vi "RANGE Grab Bank Data.vi"(0 "DAQ Data In in":T4={"Meter 1"={"Meter Size"=0.0, "DAQ Output (Voltage)"=0.0, "Reference (Voltage)"=0.0, "Meter Present"=FALSE, "Meter Visa"="COM3", "Gas Type"="12", "SLPM Error @ Zero"=0.0, "Gas Mix Number"="", "Set STP Register"=FALSE, "Measurement Units"={"Software Rev"="", "Model Number"="", "Manufacturer Info"="", "Software Sub-Rev"="", "Board Rev"="", "Units of Measure Input"={"Abs. Pressure"="", "Gauge/Diff. Press."="", "Barometric Press."="", "Temperature"="", "Volume"="", "Mass"="", "Setpoint"="", "Valve Drive"="", "Totalizer"="", "Tot. Timer"="", "Tot. Avg. Flow"="", "Tot. Peak Flow"=""}}, "Data Frame Format"={"Absolute Pressure"=FALSE, "Gauge/Diff. Pressure"=FALSE, "Barometric Pressure"=FALSE, "Temperature"=FALSE, "Volumetric"=FALSE, "Mass"=FALSE, "Setpoint"=FALSE, "Valve Drive"=FALSE, "Totalizer"=FALSE, "Totalizer Timer"=FALSE, "Totalizer Average Flow"=FALSE, "Totalizer Peak Flow"=FALSE, "Gas Selected"=FALSE, "Tot. Timer Format"=0}}, "Meter 2"={"Meter Size"=0.0, "DAQ Output (Voltage)"=0.0, "Reference (Voltage)"=0.0, "Meter Present"=FALSE, "Meter Visa"="COM3", "Gas Type"="12", "SLPM Error @ Zero"=0.0, "Gas Mix Number"="", "Set STP Register"=FALSE, "Measurement Units"={"Software Rev"="", "Model Number"="", "Manufacturer Info"="", "Software Sub-Rev"="", "Board Rev"="", "Units of Measure Input"={"Abs. Pressure"="", "Gauge/Diff. Press."="", "Barometric Press."="", "Temperature"="", "Volume"="", "Mass"="", "Setpoint"="", "Valve Drive"="", "Totalizer"="", "Tot. Timer"="", "Tot. Avg. Flow"="", "Tot. Peak Flow"=""}}, "Data Frame Format"={"Absolute Pressure"=FALSE, "Gauge/Diff. Pressure"=FALSE, "Barometric Pressure"=FALSE, "Temperature"=FALSE, "Volumetric"=FALSE, "Mass"=FALSE, "Setpoint"=FALSE, "Valve Drive"=FALSE, "Totalizer"=FALSE, "Totalizer Timer"=FALSE, "Totalizer Average Flow"=FALSE, "Totalizer Peak Flow"=FALSE, "Gas Selected"=FALSE, "Tot. Timer Format"=0}}, "Meter 3"={"Meter Size"=0.0, "DAQ Output (Voltage)"=0.0, "Reference (Voltage)"=0.0, "Meter Present"=FALSE, "Meter Visa"="COM3", "Gas Type"="12", "SLPM Error @ Zero"=0.0, "Gas Mix Number"="", "Set STP Register"=FALSE, "Measurement Units"={"Software Rev"="", "Model Number"="", "Manufacturer Info"="", "Software Sub-Rev"="", "Board Rev"="", "Units of Measure Input"={"Abs. Pressure"="", "Gauge/Diff. Press."="", "Barometric Press."="", "Temperature"="", "Volume"="", "Mass"="", "Setpoint"="", "Valve Drive"="", "Totalizer"="", "Tot. Timer"="", "Tot. Avg. Flow"="", "Tot. Peak Flow"=""}}, "Data Frame Format"={"Absolute Pressure"=FALSE, "Gauge/Diff. Pressure"=FALSE, "Barometric Pressure"=FALSE, "Temperature"=FALSE, "Volumetric"=FALSE, "Mass"=FALSE, "Setpoint"=FALSE, "Valve Drive"=FALSE, "Totalizer"=FALSE, "Totalizer Timer"=FALSE, "Totalizer Average Flow"=FALSE, "Totalizer Peak Flow"=FALSE, "Gas Selected"=FALSE, "Tot. Timer Format"=0}}, "Meter 4"={"Meter Size"=0.0, "DAQ Output (Voltage)"=0.0, "Reference (Voltage)"=0.0, "Meter Present"=FALSE, "Meter Visa"="COM3", "Gas Type"="12", "SLPM Error @ Zero"=0.0, "Gas Mix Number"="", "Set STP Register"=FALSE, "Measurement Units"={"Software Rev"="", "Model Number"="", "Manufacturer Info"="", "Software Sub-Rev"="", "Board Rev"="", "Units of Measure Input"={"Abs. Pressure"="", "Gauge/Diff. Press."="", "Barometric Press."="", "Temperature"="", "Volume"="", "Mass"="", "Setpoint"="", "Valve Drive"="", "Totalizer"="", "Tot. Timer"="", "Tot. Avg. Flow"="", "Tot. Peak Flow"=""}}, "Data Frame Format"={"Absolute Pressure"=FALSE, "Gauge/Diff. Pressure"=FALSE, "Barometric Pressure"=FALSE, "Temperature"=FALSE, "Volumetric"=FALSE, "Mass"=FALSE, "Setpoint"=FALSE, "Valve Drive"=FALSE, "Totalizer"=FALSE, "Totalizer Timer"=FALSE, "Totalizer Average Flow"=FALSE, "Totalizer Peak Flow"=FALSE, "Gas Selected"=FALSE, "Tot. Timer Format"=0}}, "Meter 5"={"Meter Size"=0.0, "DAQ Output (Voltage)"=0.0, "Reference (Voltage)"=0.0, "Meter Present"=FALSE, "Meter Visa"="COM3", "Gas Type"="12", "SLPM Error @ Zero"=0.0, "Gas Mix Number"="", "Set STP Register"=FALSE, "Measurement Units"={"Software Rev"="", "Model Number"="", "Manufacturer Info"="", "Software Sub-Rev"="", "Board Rev"="", "Units of Measure Input"={"Abs. Pressure"="", "Gauge/Diff. Press."="", "Barometric Press."="", "Temperature"="", "Volume"="", "Mass"="", "Setpoint"="", "Valve Drive"="", "Totalizer"="", "Tot. Timer"="", "Tot. Avg. Flow"="", "Tot. Peak Flow"=""}}, "Data Frame Format"={"Absolute Pressure"=FALSE, "Gauge/Diff. Pressure"=FALSE, "Barometric Pressure"=FALSE, "Temperature"=FALSE, "Volumetric"=FALSE, "Mass"=FALSE, "Setpoint"=FALSE, "Valve Drive"=FALSE, "Totalizer"=FALSE, "Totalizer Timer"=FALSE, "Totalizer Average Flow"=FALSE, "Totalizer Peak Flow"=FALSE, "Gas Selected"=FALSE, "Tot. Timer Format"=0}}, "Meter 6"={"Meter Size"=0.0, "DAQ Output (Voltage)"=0.0, "Reference (Voltage)"=0.0, "Meter Present"=FALSE, "Meter Visa"="COM3", "Gas Type"="12", "SLPM Error @ Zero"=0.0, "Gas Mix Number"="", "Set STP Register"=FALSE, "Measurement Units"={"Software Rev"="", "Model Number"="", "Manufacturer Info"="", "Software Sub-Rev"="", "Board Rev"="", "Units of Measure Input"={"Abs. Pressure"="", "Gauge/Diff. Press."="", "Barometric Press."="", "Temperature"="", "Volume"="", "Mass"="", "Setpoint"="", "Valve Drive"="", "Totalizer"="", "Tot. Timer"="", "Tot. Avg. Flow"="", "Tot. Peak Flow"=""}}, "Data Frame Format"={"Absolute Pressure"=FALSE, "Gauge/Diff. Pressure"=FALSE, "Barometric Pressure"=FALSE, "Temperature"=FALSE, "Volumetric"=FALSE, "Mass"=FALSE, "Setpoint"=FALSE, "Valve Drive"=FALSE, "Totalizer"=FALSE, "Totalizer Timer"=FALSE, "Totalizer Average Flow"=FALSE, "Totalizer Peak Flow"=FALSE, "Gas Selected"=FALSE, "Tot. Timer Format"=0}}, "Meter Bank 1"={"Flow Rate (BTU/HR)"=0.0, "ANSI Average (BTU/HR)"=0.0, "Panel Data"={"Meter Type (Gas)"="", "Heating Value (BTU/ft³)"=0.0, "Ft³ / Hr (SCFH)"=0.0, "15 Second Average (BTU/HR)"=0.0, "30 Second Average (BTU/HR)"=0.0, "Mass Flow"=0.0, "Vol. Flow"=0.0, "Gas Temperature"=0.0, "Gas Pressure"=0.0, "Tot.Flow"=0.0}, "Meter ID"="", "ANSI Rate"={"Array 1"=[], "Array 3"=[], "Array 2"=[], "Start ANSI"=FALSE, "ANSI Start Time"=0.0, "Restart ANSI"=FALSE, "15 Min ANSI Avg (BTU/hr)"=0.0, "20 Min ANSI Avg (BTU/hr)"=0.0, "25 Min ANSI Avg (BTU/hr)"=0.0, "Absolute Pressure"=0.0, "Gas Temperature"=0.0, "Volumetric Flow Rate"=0.0, "Mass Flow Rate"=0.0, "Array 4"=[], "Array 5"=[], "Gas Rate"=0.0, "15 Min Pres Avg (PSIA)"=0.0, "20 Min Pres Avg (PSIA)"=0.0, "25 Min Pres Avg (PSIA)"=0.0, "15 Min Temp Avg (°F) "=0.0, "20 Min Temp Avg (°F)"=0.0, "25 Min Temp Avg (°F)"=0.0, "15 Min Uncorrected Avg (CFH)"=0.0, "20 Min Uncorrected Avg (CFH)"=0.0, "25 Min Uncorrected Avg (CFH)"=0.0, "15 Min Corrected Avg (SCFH)"=0.0, "20 Min Corrected Avg (SCFH)"=0.0, "25 Min Corrected Avg (SCFH)"=0.0, "15 Min Complete"=FALSE, "20 Min Complete"=FALSE, "25 Min Complete"=FALSE, "Heating Value (BTU/ft³)"=0.0, "CO CO2 15 Min"=[], "CO CO2 20 Min"=[], "CO CO2 25 Min"=[], "CO CO2 Real Time"=[]}}, "Meter Bank 2"={"Flow Rate (BTU/HR)"=0.0, "ANSI Average (BTU/HR)"=0.0, "Panel Data"={"Meter Type (Gas)"="", "Heating Value (BTU/ft³)"=0.0, "Ft³ / Hr (SCFH)"=0.0, "15 Second Average (BTU/HR)"=0.0, "30 Second Average (BTU/HR)"=0.0, "Mass Flow"=0.0, "Vol. Flow"=0.0, "Gas Temperature"=0.0, "Gas Pressure"=0.0, "Tot.Flow"=0.0}, "Meter ID"="", "ANSI Rate"={"Array 1"=[], "Array 3"=[], "Array 2"=[], "Start ANSI"=FALSE, "ANSI Start Time"=0.0, "Restart ANSI"=FALSE, "15 Min ANSI Avg (BTU/hr)"=0.0, "20 Min ANSI Avg (BTU/hr)"=0.0, "25 Min ANSI Avg (BTU/hr)"=0.0, "Absolute Pressure"=0.0, "Gas Temperature"=0.0, "Volumetric Flow Rate"=0.0, "Mass Flow Rate"=0.0, "Array 4"=[], "Array 5"=[], "Gas Rate"=0.0, "15 Min Pres Avg (PSIA)"=0.0, "20 Min Pres Avg (PSIA)"=0.0, "25 Min Pres Avg (PSIA)"=0.0, "15 Min Temp Avg (°F) "=0.0, "20 Min Temp Avg (°F)"=0.0, "25 Min Temp Avg (°F)"=0.0, "15 Min Uncorrected Avg (CFH)"=0.0, "20 Min Uncorrected Avg (CFH)"=0.0, "25 Min Uncorrected Avg (CFH)"=0.0, "15 Min Corrected Avg (SCFH)"=0.0, "20 Min Corrected Avg (SCFH)"=0.0, "25 Min Corrected Avg (SCFH)"=0.0, "15 Min Complete"=FALSE, "20 Min Complete"=FALSE, "25 Min Complete"=FALSE, "Heating Value (BTU/ft³)"=0.0, "CO CO2 15 Min"=[], "CO CO2 20 Min"=[], "CO CO2 25 Min"=[], "CO CO2 Real Time"=[]}}, "Meter Bank 3"={"Flow Rate (BTU/HR)"=0.0, "ANSI Average (BTU/HR)"=0.0, "Panel Data"={"Meter Type (Gas)"="", "Heating Value (BTU/ft³)"=0.0, "Ft³ / Hr (SCFH)"=0.0, "15 Second Average (BTU/HR)"=0.0, "30 Second Average (BTU/HR)"=0.0, "Mass Flow"=0.0, "Vol. Flow"=0.0, "Gas Temperature"=0.0, "Gas Pressure"=0.0, "Tot.Flow"=0.0}, "Meter ID"="", "ANSI Rate"={"Array 1"=[], "Array 3"=[], "Array 2"=[], "Start ANSI"=FALSE, "ANSI Start Time"=0.0, "Restart ANSI"=FALSE, "15 Min ANSI Avg (BTU/hr)"=0.0, "20 Min ANSI Avg (BTU/hr)"=0.0, "25 Min ANSI Avg (BTU/hr)"=0.0, "Absolute Pressure"=0.0, "Gas Temperature"=0.0, "Volumetric Flow Rate"=0.0, "Mass Flow Rate"=0.0, "Array 4"=[], "Array 5"=[], "Gas Rate"=0.0, "15 Min Pres Avg (PSIA)"=0.0, "20 Min Pres Avg (PSIA)"=0.0, "25 Min Pres Avg (PSIA)"=0.0, "15 Min Temp Avg (°F) "=0.0, "20 Min Temp Avg (°F)"=0.0, "25 Min Temp Avg (°F)"=0.0, "15 Min Uncorrected Avg (CFH)"=0.0, "20 Min Uncorrected Avg (CFH)"=0.0, "25 Min Uncorrected Avg (CFH)"=0.0, "15 Min Corrected Avg (SCFH)"=0.0, "20 Min Corrected Avg (SCFH)"=0.0, "25 Min Corrected Avg (SCFH)"=0.0, "15 Min Complete"=FALSE, "20 Min Complete"=FALSE, "25 Min Complete"=FALSE, "Heating Value (BTU/ft³)"=0.0, "CO CO2 15 Min"=[], "CO CO2 20 Min"=[], "CO CO2 25 Min"=[], "CO CO2 Real Time"=[]}}, "Threshold Voltage (NI DAQ)"=0.0, "Use RS232 Data Collection"=FALSE, "Use Auto Switching"=FALSE}, 1 "Meter Number":T13, 2 "Tot.Flow (Liters) Bank 2":dbl, 3 "Use Mass Flow Unit Converter?":bool, 5 "Meter Select":T3, 7 "Tot.Flow (Liters) Bank 1":dbl, 9 "Meter Select 2":T1, 11 "error in (no error)":errorcluster, 12 "Meter Select 3":T2, 13 "Tot.Flow (Liters) Bank 3":dbl) -> (4 "DAQ Data In out":T4={"Meter 1"={"Meter Size"=0.0, "DAQ Output (Voltage)"=0.0, "Reference (Voltage)"=0.0, "Meter Present"=FALSE, "Meter Visa"="COM3", "Gas Type"="12", "SLPM Error @ Zero"=0.0, "Gas Mix Number"="", "Set STP Register"=FALSE, "Measurement Units"={"Software Rev"="", "Model Number"="", "Manufacturer Info"="", "Software Sub-Rev"="", "Board Rev"="", "Units of Measure Input"={"Abs. Pressure"="", "Gauge/Diff. Press."="", "Barometric Press."="", "Temperature"="", "Volume"="", "Mass"="", "Setpoint"="", "Valve Drive"="", "Totalizer"="", "Tot. Timer"="", "Tot. Avg. Flow"="", "Tot. Peak Flow"=""}}, "Data Frame Format"={"Absolute Pressure"=FALSE, "Gauge/Diff. Pressure"=FALSE, "Barometric Pressure"=FALSE, "Temperature"=FALSE, "Volumetric"=FALSE, "Mass"=FALSE, "Setpoint"=FALSE, "Valve Drive"=FALSE, "Totalizer"=FALSE, "Totalizer Timer"=FALSE, "Totalizer Average Flow"=FALSE, "Totalizer Peak Flow"=FALSE, "Gas Selected"=FALSE, "Tot. Timer Format"=0}}, "Meter 2"={"Meter Size"=0.0, "DAQ Output (Voltage)"=0.0, "Reference (Voltage)"=0.0, "Meter Present"=FALSE, "Meter Visa"="COM3", "Gas Type"="12", "SLPM Error @ Zero"=0.0, "Gas Mix Number"="", "Set STP Register"=FALSE, "Measurement Units"={"Software Rev"="", "Model Number"="", "Manufacturer Info"="", "Software Sub-Rev"="", "Board Rev"="", "Units of Measure Input"={"Abs. Pressure"="", "Gauge/Diff. Press."="", "Barometric Press."="", "Temperature"="", "Volume"="", "Mass"="", "Setpoint"="", "Valve Drive"="", "Totalizer"="", "Tot. Timer"="", "Tot. Avg. Flow"="", "Tot. Peak Flow"=""}}, "Data Frame Format"={"Absolute Pressure"=FALSE, "Gauge/Diff. Pressure"=FALSE, "Barometric Pressure"=FALSE, "Temperature"=FALSE, "Volumetric"=FALSE, "Mass"=FALSE, "Setpoint"=FALSE, "Valve Drive"=FALSE, "Totalizer"=FALSE, "Totalizer Timer"=FALSE, "Totalizer Average Flow"=FALSE, "Totalizer Peak Flow"=FALSE, "Gas Selected"=FALSE, "Tot. Timer Format"=0}}, "Meter 3"={"Meter Size"=0.0, "DAQ Output (Voltage)"=0.0, "Reference (Voltage)"=0.0, "Meter Present"=FALSE, "Meter Visa"="COM3", "Gas Type"="12", "SLPM Error @ Zero"=0.0, "Gas Mix Number"="", "Set STP Register"=FALSE, "Measurement Units"={"Software Rev"="", "Model Number"="", "Manufacturer Info"="", "Software Sub-Rev"="", "Board Rev"="", "Units of Measure Input"={"Abs. Pressure"="", "Gauge/Diff. Press."="", "Barometric Press."="", "Temperature"="", "Volume"="", "Mass"="", "Setpoint"="", "Valve Drive"="", "Totalizer"="", "Tot. Timer"="", "Tot. Avg. Flow"="", "Tot. Peak Flow"=""}}, "Data Frame Format"={"Absolute Pressure"=FALSE, "Gauge/Diff. Pressure"=FALSE, "Barometric Pressure"=FALSE, "Temperature"=FALSE, "Volumetric"=FALSE, "Mass"=FALSE, "Setpoint"=FALSE, "Valve Drive"=FALSE, "Totalizer"=FALSE, "Totalizer Timer"=FALSE, "Totalizer Average Flow"=FALSE, "Totalizer Peak Flow"=FALSE, "Gas Selected"=FALSE, "Tot. Timer Format"=0}}, "Meter 4"={"Meter Size"=0.0, "DAQ Output (Voltage)"=0.0, "Reference (Voltage)"=0.0, "Meter Present"=FALSE, "Meter Visa"="COM3", "Gas Type"="12", "SLPM Error @ Zero"=0.0, "Gas Mix Number"="", "Set STP Register"=FALSE, "Measurement Units"={"Software Rev"="", "Model Number"="", "Manufacturer Info"="", "Software Sub-Rev"="", "Board Rev"="", "Units of Measure Input"={"Abs. Pressure"="", "Gauge/Diff. Press."="", "Barometric Press."="", "Temperature"="", "Volume"="", "Mass"="", "Setpoint"="", "Valve Drive"="", "Totalizer"="", "Tot. Timer"="", "Tot. Avg. Flow"="", "Tot. Peak Flow"=""}}, "Data Frame Format"={"Absolute Pressure"=FALSE, "Gauge/Diff. Pressure"=FALSE, "Barometric Pressure"=FALSE, "Temperature"=FALSE, "Volumetric"=FALSE, "Mass"=FALSE, "Setpoint"=FALSE, "Valve Drive"=FALSE, "Totalizer"=FALSE, "Totalizer Timer"=FALSE, "Totalizer Average Flow"=FALSE, "Totalizer Peak Flow"=FALSE, "Gas Selected"=FALSE, "Tot. Timer Format"=0}}, "Meter 5"={"Meter Size"=0.0, "DAQ Output (Voltage)"=0.0, "Reference (Voltage)"=0.0, "Meter Present"=FALSE, "Meter Visa"="COM3", "Gas Type"="12", "SLPM Error @ Zero"=0.0, "Gas Mix Number"="", "Set STP Register"=FALSE, "Measurement Units"={"Software Rev"="", "Model Number"="", "Manufacturer Info"="", "Software Sub-Rev"="", "Board Rev"="", "Units of Measure Input"={"Abs. Pressure"="", "Gauge/Diff. Press."="", "Barometric Press."="", "Temperature"="", "Volume"="", "Mass"="", "Setpoint"="", "Valve Drive"="", "Totalizer"="", "Tot. Timer"="", "Tot. Avg. Flow"="", "Tot. Peak Flow"=""}}, "Data Frame Format"={"Absolute Pressure"=FALSE, "Gauge/Diff. Pressure"=FALSE, "Barometric Pressure"=FALSE, "Temperature"=FALSE, "Volumetric"=FALSE, "Mass"=FALSE, "Setpoint"=FALSE, "Valve Drive"=FALSE, "Totalizer"=FALSE, "Totalizer Timer"=FALSE, "Totalizer Average Flow"=FALSE, "Totalizer Peak Flow"=FALSE, "Gas Selected"=FALSE, "Tot. Timer Format"=0}}, "Meter 6"={"Meter Size"=0.0, "DAQ Output (Voltage)"=0.0, "Reference (Voltage)"=0.0, "Meter Present"=FALSE, "Meter Visa"="COM3", "Gas Type"="12", "SLPM Error @ Zero"=0.0, "Gas Mix Number"="", "Set STP Register"=FALSE, "Measurement Units"={"Software Rev"="", "Model Number"="", "Manufacturer Info"="", "Software Sub-Rev"="", "Board Rev"="", "Units of Measure Input"={"Abs. Pressure"="", "Gauge/Diff. Press."="", "Barometric Press."="", "Temperature"="", "Volume"="", "Mass"="", "Setpoint"="", "Valve Drive"="", "Totalizer"="", "Tot. Timer"="", "Tot. Avg. Flow"="", "Tot. Peak Flow"=""}}, "Data Frame Format"={"Absolute Pressure"=FALSE, "Gauge/Diff. Pressure"=FALSE, "Barometric Pressure"=FALSE, "Temperature"=FALSE, "Volumetric"=FALSE, "Mass"=FALSE, "Setpoint"=FALSE, "Valve Drive"=FALSE, "Totalizer"=FALSE, "Totalizer Timer"=FALSE, "Totalizer Average Flow"=FALSE, "Totalizer Peak Flow"=FALSE, "Gas Selected"=FALSE, "Tot. Timer Format"=0}}, "Meter Bank 1"={"Flow Rate (BTU/HR)"=0.0, "ANSI Average (BTU/HR)"=0.0, "Panel Data"={"Meter Type (Gas)"="", "Heating Value (BTU/ft³)"=0.0, "Ft³ / Hr (SCFH)"=0.0, "15 Second Average (BTU/HR)"=0.0, "30 Second Average (BTU/HR)"=0.0, "Mass Flow"=0.0, "Vol. Flow"=0.0, "Gas Temperature"=0.0, "Gas Pressure"=0.0, "Tot.Flow"=0.0}, "Meter ID"="", "ANSI Rate"={"Array 1"=[], "Array 3"=[], "Array 2"=[], "Start ANSI"=FALSE, "ANSI Start Time"=0.0, "Restart ANSI"=FALSE, "15 Min ANSI Avg (BTU/hr)"=0.0, "20 Min ANSI Avg (BTU/hr)"=0.0, "25 Min ANSI Avg (BTU/hr)"=0.0, "Absolute Pressure"=0.0, "Gas Temperature"=0.0, "Volumetric Flow Rate"=0.0, "Mass Flow Rate"=0.0, "Array 4"=[], "Array 5"=[], "Gas Rate"=0.0, "15 Min Pres Avg (PSIA)"=0.0, "20 Min Pres Avg (PSIA)"=0.0, "25 Min Pres Avg (PSIA)"=0.0, "15 Min Temp Avg (°F) "=0.0, "20 Min Temp Avg (°F)"=0.0, "25 Min Temp Avg (°F)"=0.0, "15 Min Uncorrected Avg (CFH)"=0.0, "20 Min Uncorrected Avg (CFH)"=0.0, "25 Min Uncorrected Avg (CFH)"=0.0, "15 Min Corrected Avg (SCFH)"=0.0, "20 Min Corrected Avg (SCFH)"=0.0, "25 Min Corrected Avg (SCFH)"=0.0, "15 Min Complete"=FALSE, "20 Min Complete"=FALSE, "25 Min Complete"=FALSE, "Heating Value (BTU/ft³)"=0.0, "CO CO2 15 Min"=[], "CO CO2 20 Min"=[], "CO CO2 25 Min"=[], "CO CO2 Real Time"=[]}}, "Meter Bank 2"={"Flow Rate (BTU/HR)"=0.0, "ANSI Average (BTU/HR)"=0.0, "Panel Data"={"Meter Type (Gas)"="", "Heating Value (BTU/ft³)"=0.0, "Ft³ / Hr (SCFH)"=0.0, "15 Second Average (BTU/HR)"=0.0, "30 Second Average (BTU/HR)"=0.0, "Mass Flow"=0.0, "Vol. Flow"=0.0, "Gas Temperature"=0.0, "Gas Pressure"=0.0, "Tot.Flow"=0.0}, "Meter ID"="", "ANSI Rate"={"Array 1"=[], "Array 3"=[], "Array 2"=[], "Start ANSI"=FALSE, "ANSI Start Time"=0.0, "Restart ANSI"=FALSE, "15 Min ANSI Avg (BTU/hr)"=0.0, "20 Min ANSI Avg (BTU/hr)"=0.0, "25 Min ANSI Avg (BTU/hr)"=0.0, "Absolute Pressure"=0.0, "Gas Temperature"=0.0, "Volumetric Flow Rate"=0.0, "Mass Flow Rate"=0.0, "Array 4"=[], "Array 5"=[], "Gas Rate"=0.0, "15 Min Pres Avg (PSIA)"=0.0, "20 Min Pres Avg (PSIA)"=0.0, "25 Min Pres Avg (PSIA)"=0.0, "15 Min Temp Avg (°F) "=0.0, "20 Min Temp Avg (°F)"=0.0, "25 Min Temp Avg (°F)"=0.0, "15 Min Uncorrected Avg (CFH)"=0.0, "20 Min Uncorrected Avg (CFH)"=0.0, "25 Min Uncorrected Avg (CFH)"=0.0, "15 Min Corrected Avg (SCFH)"=0.0, "20 Min Corrected Avg (SCFH)"=0.0, "25 Min Corrected Avg (SCFH)"=0.0, "15 Min Complete"=FALSE, "20 Min Complete"=FALSE, "25 Min Complete"=FALSE, "Heating Value (BTU/ft³)"=0.0, "CO CO2 15 Min"=[], "CO CO2 20 Min"=[], "CO CO2 25 Min"=[], "CO CO2 Real Time"=[]}}, "Meter Bank 3"={"Flow Rate (BTU/HR)"=0.0, "ANSI Average (BTU/HR)"=0.0, "Panel Data"={"Meter Type (Gas)"="", "Heating Value (BTU/ft³)"=0.0, "Ft³ / Hr (SCFH)"=0.0, "15 Second Average (BTU/HR)"=0.0, "30 Second Average (BTU/HR)"=0.0, "Mass Flow"=0.0, "Vol. Flow"=0.0, "Gas Temperature"=0.0, "Gas Pressure"=0.0, "Tot.Flow"=0.0}, "Meter ID"="", "ANSI Rate"={"Array 1"=[], "Array 3"=[], "Array 2"=[], "Start ANSI"=FALSE, "ANSI Start Time"=0.0, "Restart ANSI"=FALSE, "15 Min ANSI Avg (BTU/hr)"=0.0, "20 Min ANSI Avg (BTU/hr)"=0.0, "25 Min ANSI Avg (BTU/hr)"=0.0, "Absolute Pressure"=0.0, "Gas Temperature"=0.0, "Volumetric Flow Rate"=0.0, "Mass Flow Rate"=0.0, "Array 4"=[], "Array 5"=[], "Gas Rate"=0.0, "15 Min Pres Avg (PSIA)"=0.0, "20 Min Pres Avg (PSIA)"=0.0, "25 Min Pres Avg (PSIA)"=0.0, "15 Min Temp Avg (°F) "=0.0, "20 Min Temp Avg (°F)"=0.0, "25 Min Temp Avg (°F)"=0.0, "15 Min Uncorrected Avg (CFH)"=0.0, "20 Min Uncorrected Avg (CFH)"=0.0, "25 Min Uncorrected Avg (CFH)"=0.0, "15 Min Corrected Avg (SCFH)"=0.0, "20 Min Corrected Avg (SCFH)"=0.0, "25 Min Corrected Avg (SCFH)"=0.0, "15 Min Complete"=FALSE, "20 Min Complete"=FALSE, "25 Min Complete"=FALSE, "Heating Value (BTU/ft³)"=0.0, "CO CO2 15 Min"=[], "CO CO2 20 Min"=[], "CO CO2 25 Min"=[], "CO CO2 Real Time"=[]}}, "Threshold Voltage (NI DAQ)"=0.0, "Use RS232 Data Collection"=FALSE, "Use Auto Switching"=FALSE}, 15 "error out":errorcluster)   [LabVIEW 2023]
uses:
  Type Definitions/RANGE DAQ Data Four Meters.ctl
  Type Definitions/RANGE DAQ Data.ctl
  Drivers/Omega FMA-1600A Series Gas Flow Meter/Type Definitions/FMA1600A Gas Type.ctl
  Drivers/Omega FMA-1600A Series Gas Flow Meter/Type Definitions/FMA1600A Units String.ctl
  Drivers/Alicat Gas Meter Driver/Sub-VIs/Units of Measure.ctl
  Drivers/Alicat Gas Meter Driver/Sub-VIs/Data Frame.ctl
  Type Definitions/RANGE GAS Data.ctl
  Type Definitions/RANGE Panel Data.ctl
  Type Definitions/RANGE ANSI Rate.ctl
  Type Definitions/Range Meter Bank.ctl
  Type Definitions/RANGE Meter Selector 1-2.ctl
  Type Definitions/RANGE Meter Selector 5-6.ctl
  Type Definitions/RANGE Meter Selector 3-4.ctl
panel:
  out "x-y 2":dbl
  out "x-y":dbl
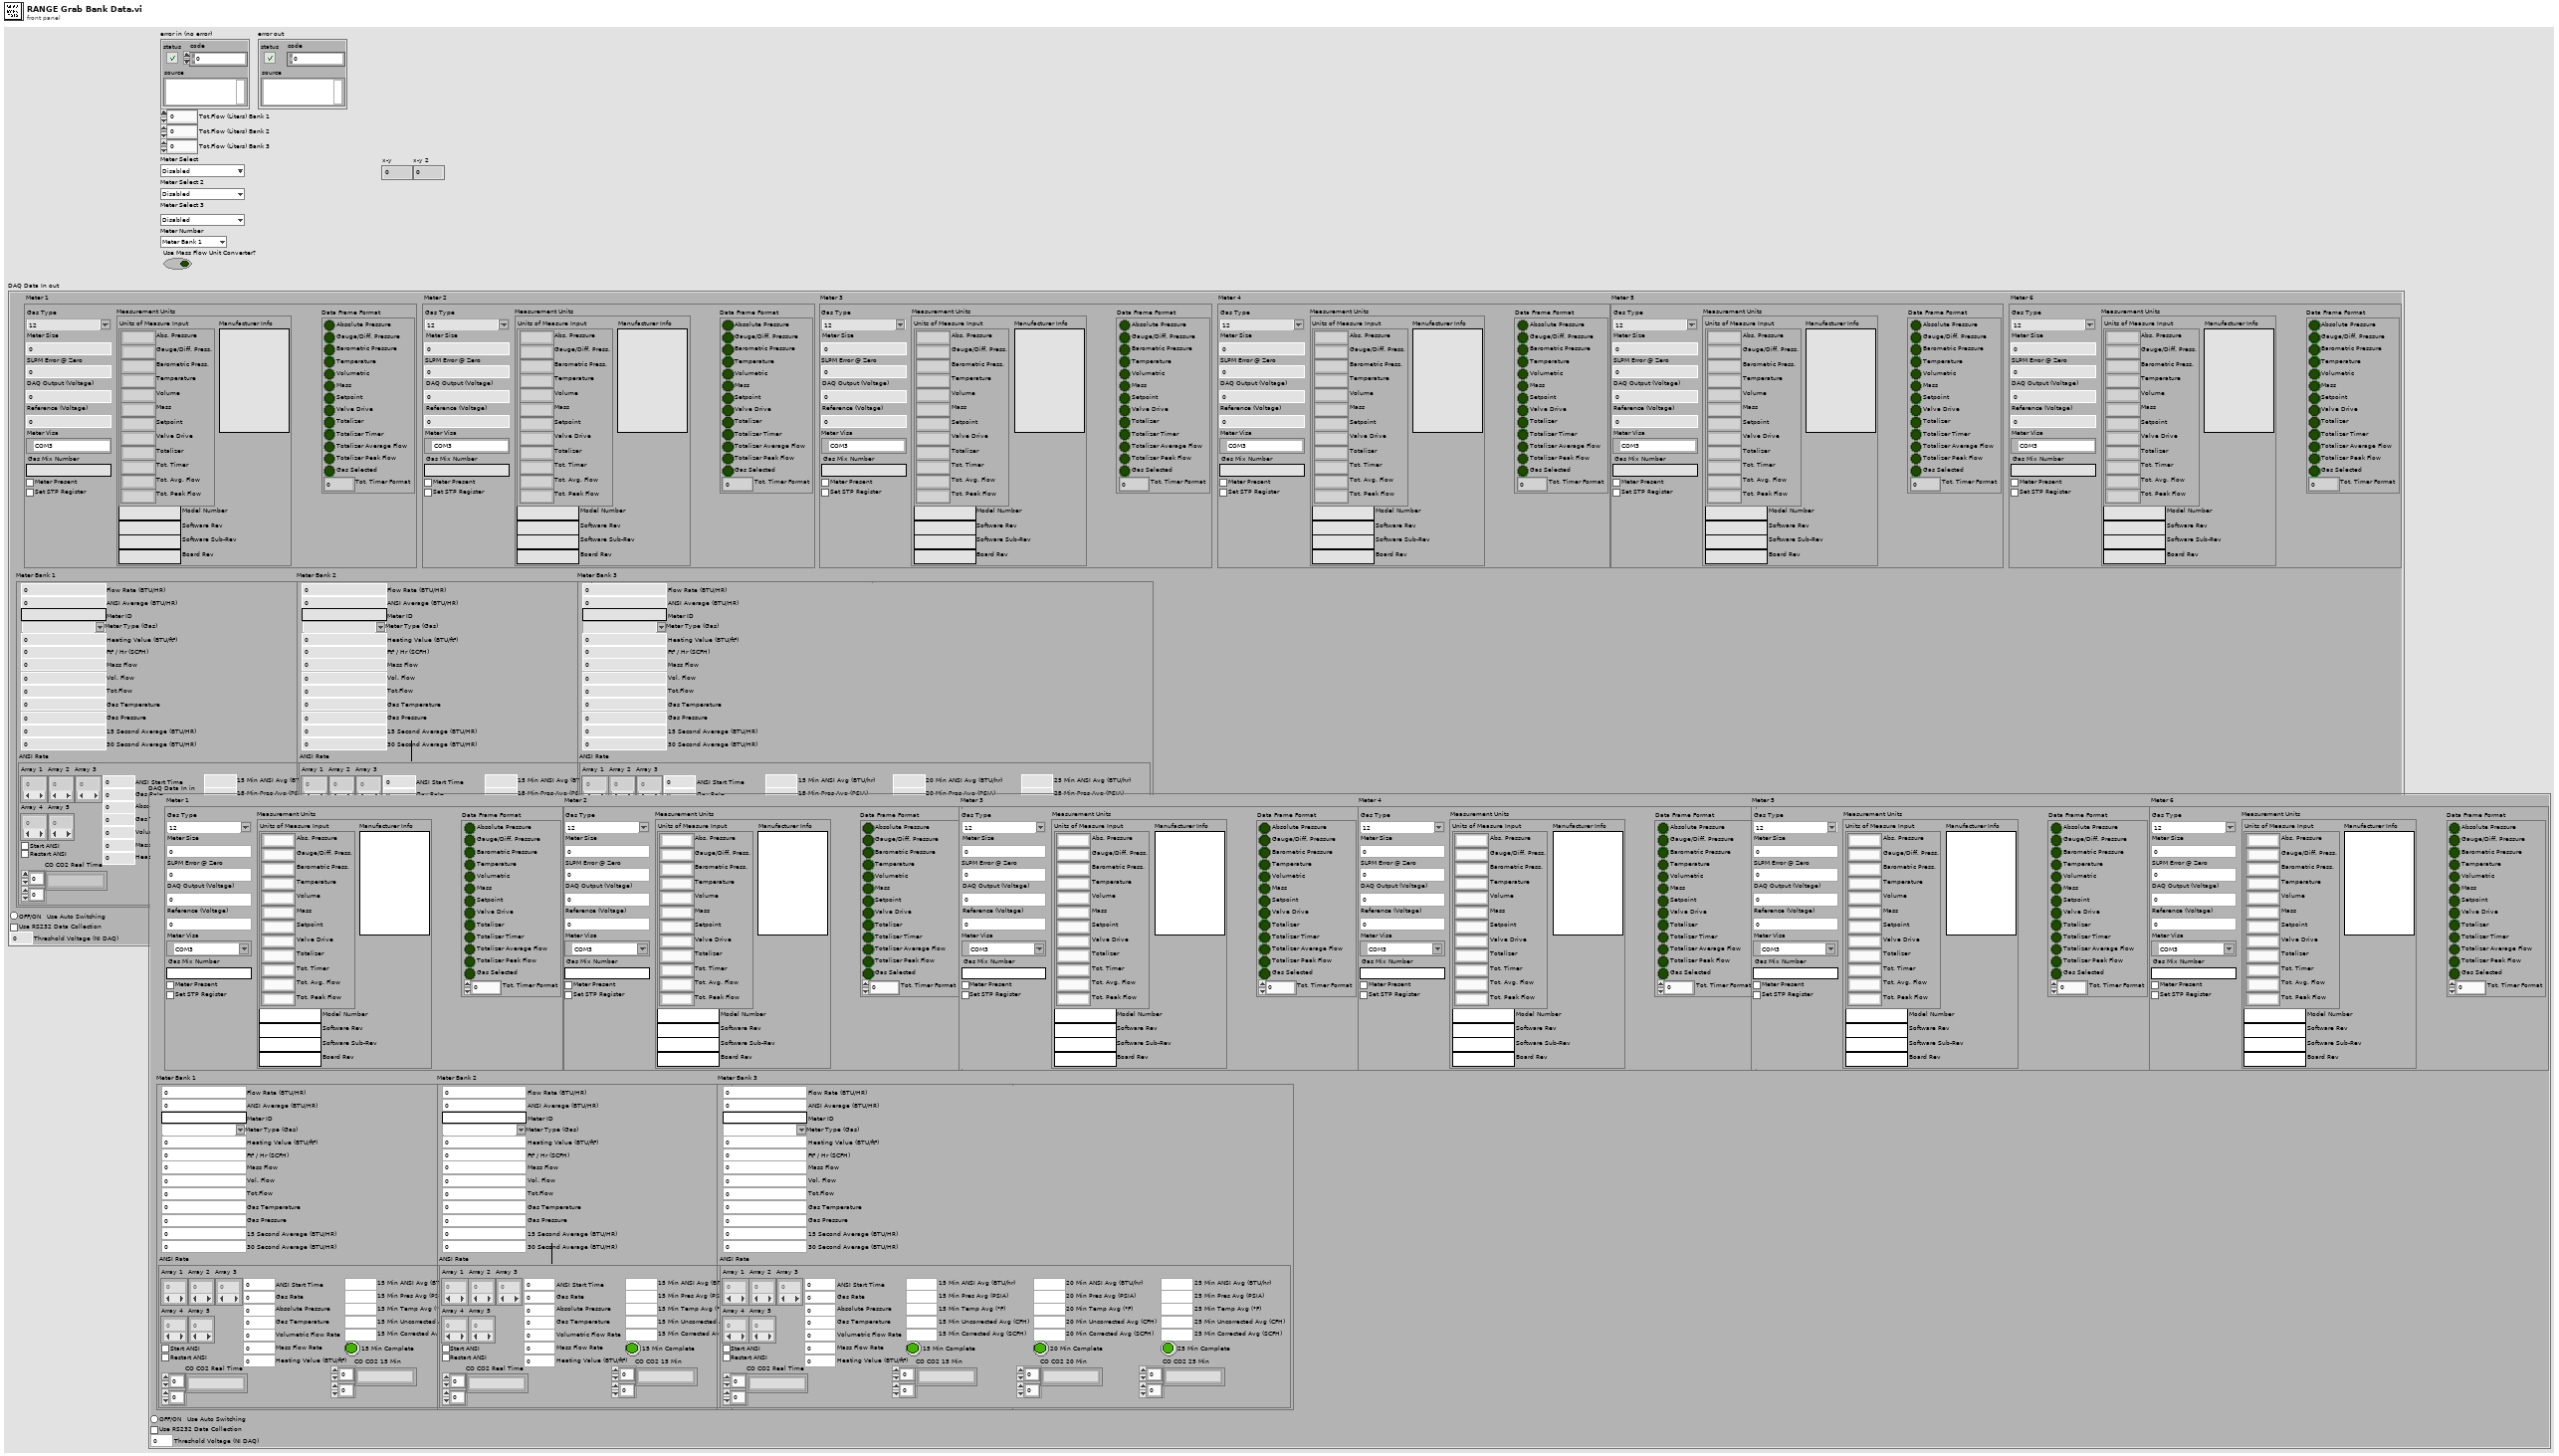
[diagram p1: front panel]
types:
  T1 = typedef "RANGE Meter Selector 3-4.ctl" = enum16{"Disabled", "Meter 3", "Meter 4", "Auto"}
  T2 = typedef "RANGE Meter Selector 5-6.ctl" = enum16{"Disabled", "Meter 5", "Meter 6", "Auto"}
  T3 = typedef "RANGE Meter Selector 1-2.ctl" = enum16{"Disabled", "Meter 1", "Meter 2", "Auto"}
  T4 = typedef "RANGE DAQ Data Four Meters.ctl" = cluster{"Meter 1":T5, "Meter 2":T5, "Meter 3":T5, "Meter 4":T5, "Meter 5":T5, "Meter 6":T5, "Meter Bank 1":T10, "Meter Bank 2":T10, "Meter Bank 3":T10, "Threshold Voltage (NI DAQ)":dbl, "Use RS232 Data Collection":bool, "Use Auto Switching":bool}
  T5 = typedef "RANGE DAQ Data.ctl" = cluster{"Meter Size":dbl, "DAQ Output (Voltage)":dbl, "Reference (Voltage)":dbl, "Meter Present":bool, "Meter Visa":refnum<visa-resource-name>, "Gas Type":T6, "SLPM Error @ Zero":dbl, "Gas Mix Number":string, "Set STP Register":bool, "Measurement Units":T7, "Data Frame Format":T9}
  T6 = typedef "FMA1600A Gas Type.ctl" = string
  T7 = typedef "FMA1600A Units String.ctl" = cluster{"Software Rev":string, "Model Number":string, "Manufacturer Info":string, "Software Sub-Rev":string, "Board Rev":string, "Units of Measure Input":T8}
  T8 = typedef "Units of Measure.ctl" = cluster{"Abs. Pressure":string, "Gauge/Diff. Press.":string, "Barometric Press.":string, "Temperature":string, "Volume":string, "Mass":string, "Setpoint":string, "Valve Drive":string, "Totalizer":string, "Tot. Timer":string, "Tot. Avg. Flow":string, "Tot. Peak Flow":string}
  T9 = typedef "Data Frame.ctl" = cluster{"Absolute Pressure":bool, "Gauge/Diff. Pressure":bool, "Barometric Pressure":bool, "Temperature":bool, "Volumetric":bool, "Mass":bool, "Setpoint":bool, "Valve Drive":bool, "Totalizer":bool, "Totalizer Timer":bool, "Totalizer Average Flow":bool, "Totalizer Peak Flow":bool, "Gas Selected":bool, "Tot. Timer Format":u16}
  T10 = typedef "RANGE GAS Data.ctl" = cluster{"Flow Rate (BTU/HR)":dbl, "ANSI Average (BTU/HR)":dbl, "Panel Data":T11, "Meter ID":string, "ANSI Rate":T12}
  T11 = typedef "RANGE Panel Data.ctl" = cluster{"Meter Type (Gas)":T6, "Heating Value (BTU/ft³)":dbl, "Ft³ / Hr (SCFH)":dbl, "15 Second Average (BTU/HR)":dbl, "30 Second Average (BTU/HR)":dbl, "Mass Flow":dbl, "Vol. Flow":dbl, "Gas Temperature":dbl, "Gas Pressure":dbl, "Tot.Flow":dbl}
  T12 = typedef "RANGE ANSI Rate.ctl" = cluster{"Array 1":dbl[], "Array 3":dbl[], "Array 2":dbl[], "Start ANSI":bool, "ANSI Start Time":dbl, "Restart ANSI":bool, "15 Min ANSI Avg (BTU/hr)":dbl, "20 Min ANSI Avg (BTU/hr)":dbl, "25 Min ANSI Avg (BTU/hr)":dbl, "Absolute Pressure":dbl, "Gas Temperature":dbl, "Volumetric Flow Rate":dbl, "Mass Flow Rate":dbl, "Array 4":dbl[], "Array 5":dbl[], "Gas Rate":dbl, "15 Min Pres Avg (PSIA)":dbl, "20 Min Pres Avg (PSIA)":dbl, "25 Min Pres Avg (PSIA)":dbl, "15 Min Temp Avg (°F) ":dbl, "20 Min Temp Avg (°F)":dbl, "25 Min Temp Avg (°F)":dbl, "15 Min Uncorrected Avg (CFH)":dbl, "20 Min Uncorrected Avg (CFH)":dbl, "25 Min Uncorrected Avg (CFH)":dbl, "15 Min Corrected Avg (SCFH)":dbl, "20 Min Corrected Avg (SCFH)":dbl, "25 Min Corrected Avg (SCFH)":dbl, "15 Min Complete":bool, "20 Min Complete":bool, "25 Min Complete":bool, "Heating Value (BTU/ft³)":dbl, "CO CO2 15 Min":string[][], "CO CO2 20 Min":string[][], "CO CO2 25 Min":string[][], "CO CO2 Real Time":string[][]}
  T13 = typedef "Range Meter Bank.ctl" = enum16{"Meter Bank 1", "Meter Bank 2", "Meter Bank 3"}
  T14 = typedef "Data Cluster.ctl" = cluster{"Absolute Pressure":dbl, "Gauge/Diff. Pressure":dbl, "Barometric Pressure":dbl, "Temperature":dbl, "Volumetric Flow":dbl, "Mass Flow":dbl, "Setpoint":dbl, "Valve Drive":dbl, "Totalizer":dbl, "[hr]":dbl, "[min]":dbl, "[sec]":dbl, "Totalizer Average Flow":dbl, "Totalizer Peak Flow":dbl, "Gas selected":string}
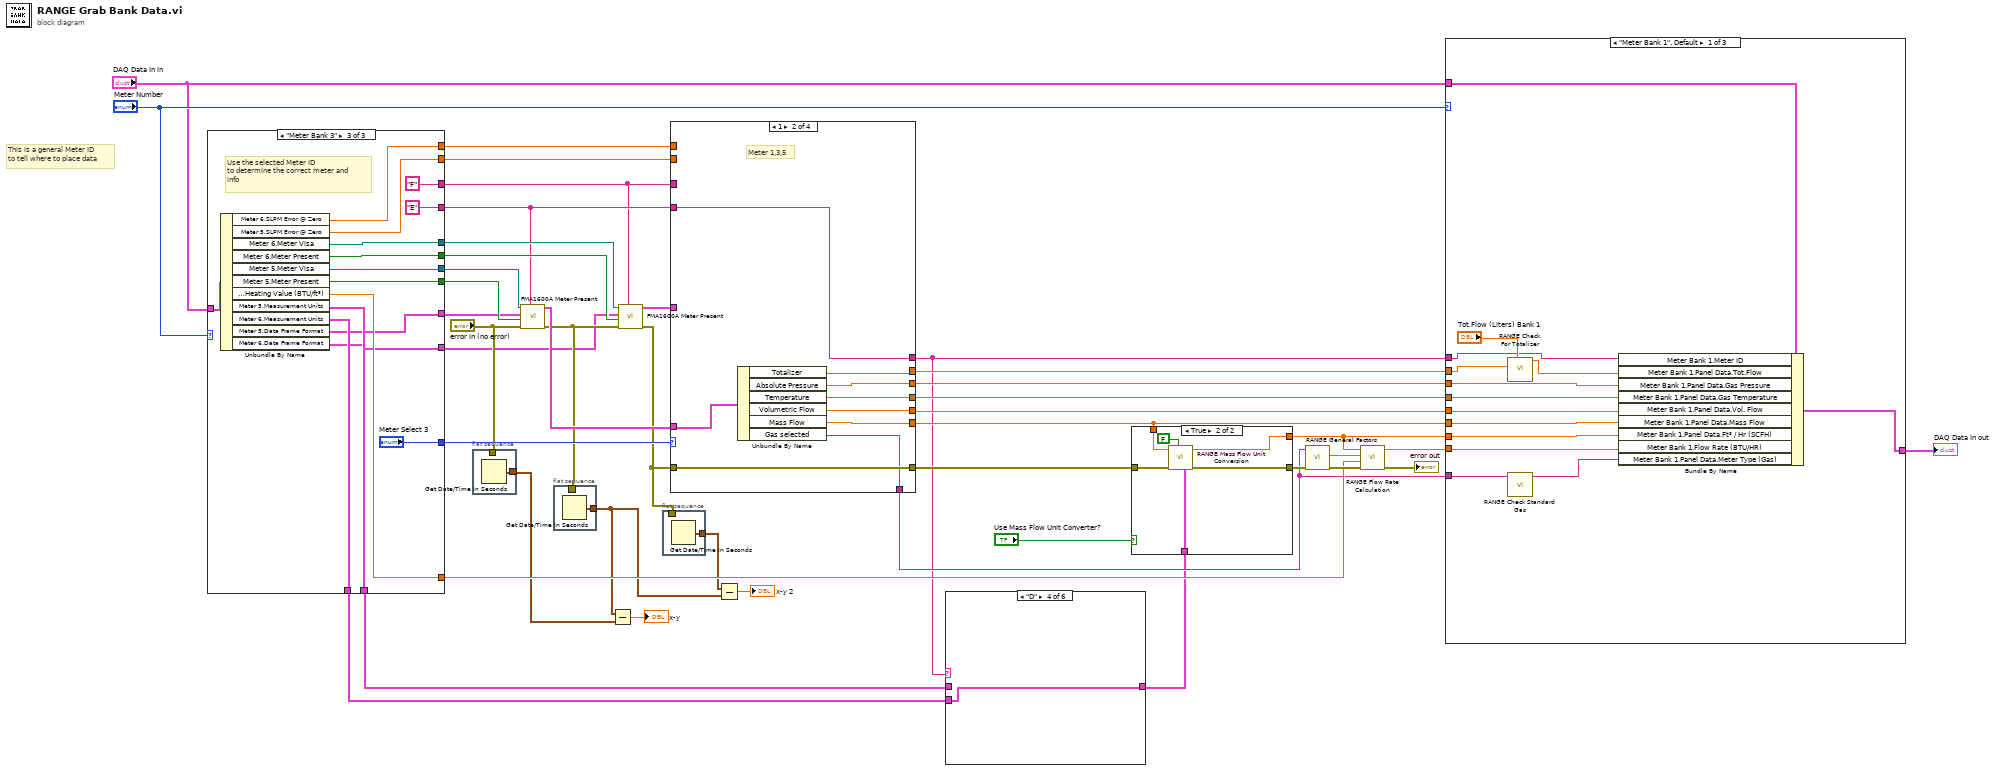
[diagram p0: block diagram]
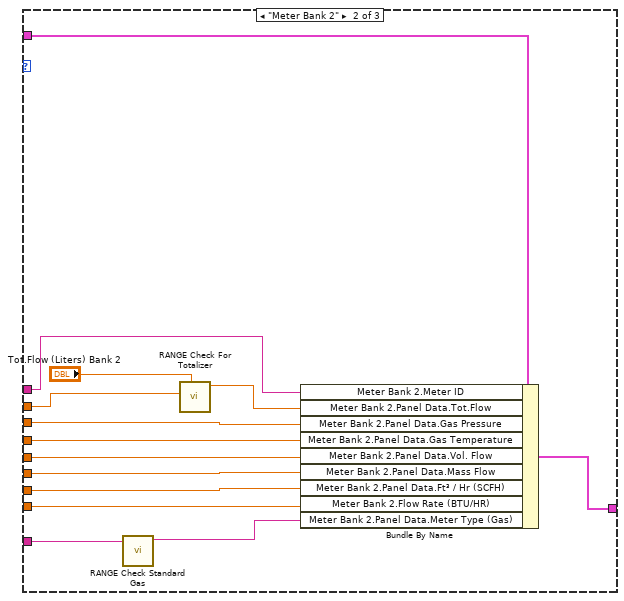
[diagram p8: hidden frame]
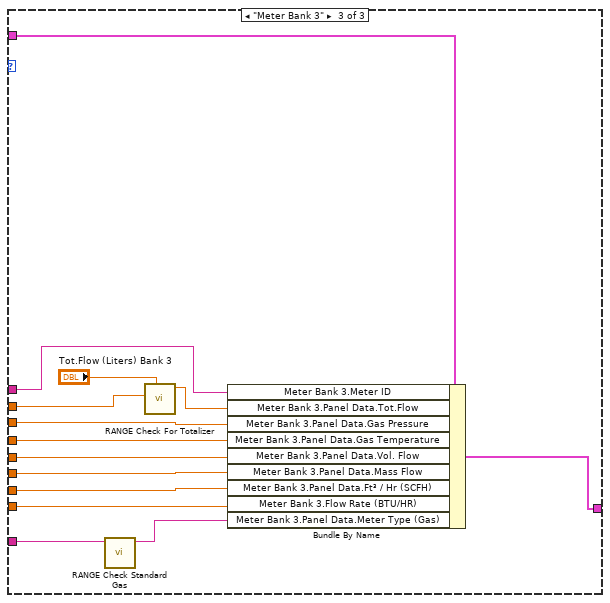
[diagram p9: hidden frame]
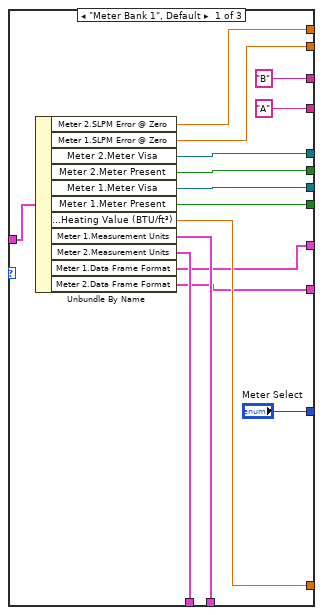
[diagram p10: hidden frame]
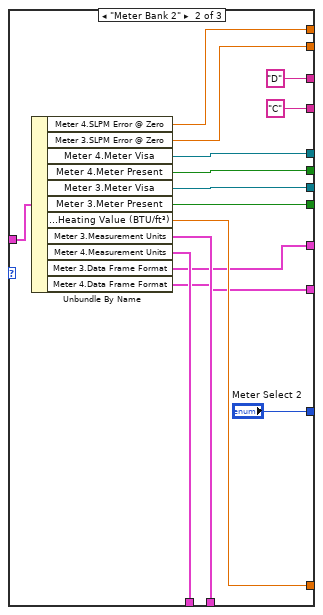
[diagram p11: hidden frame]
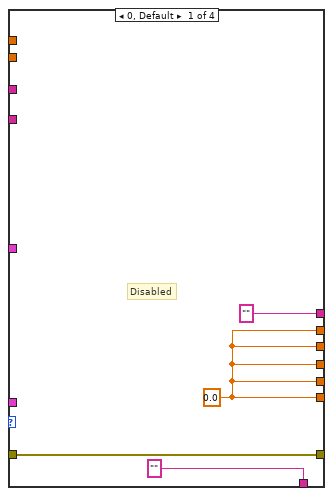
[diagram p12: hidden frame]
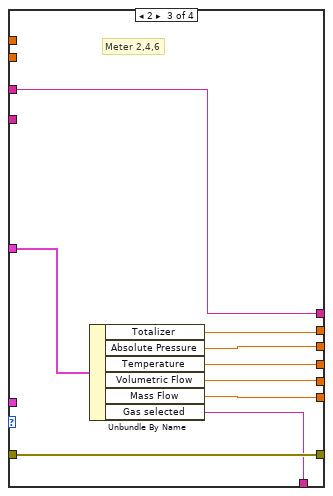
[diagram p13: hidden frame]
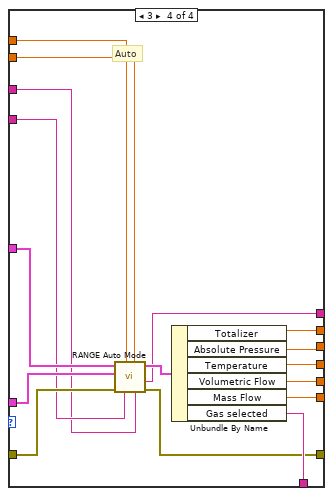
[diagram p14: hidden frame]
diagram:
  # "This is a general Meter ID\nto tell where to place data"
  n1 = case shown="\"Meter Bank 3\"" "Meter Number" {
    tunnel: ["A" ("Unit ID") "C" ("Unit ID") "E" ("Unit ID")] -> w13
    tunnel: [w57 w69 w84] -> w19
    tunnel: ["B" ("Unit ID") "D" ("Unit ID") "F" ("Unit ID")] -> w12
    tunnel: "DAQ Data In in" -> [w55 w71 w86]
    tunnel: ["Meter Select" "Meter Select 2" "Meter Select 3"] -> w41
    tunnel: [w54 w70 w85] -> w35
    tunnel: [w53 w68 w83] -> w36
    tunnel: [w52 w67 w82] -> w34
    tunnel: [w51 w66 w80] -> w21
    tunnel: [w50 w65 w81] -> w20
    tunnel: [w49 w64 w79] -> w26
    tunnel: [w47 w61 w76] -> w16
    tunnel: [w46 w62 w77] -> w17
    tunnel: [w45 w60 w75] -> w2
    tunnel: [w44 w59 w74] -> w1
    frame "Meter Bank 1", Default {
      n2 = Unbundle By Name(w55) -> ("Meter 2.SLPM Error @ Zero"=w51:dbl, "Meter 1.SLPM Error @ Zero"=w50:dbl, "Meter 2.Meter Visa"=w54:refnum<visa-resource-name>, "Meter 2.Meter Present"=w52:bool, "Meter 1.Meter Visa"=w57:refnum<visa-resource-name>, "Meter 1.Meter Present"=w53:bool, "Meter Bank 1.Panel Data.Heating Value (BTU/ft³)"=w49:dbl, "Meter 1.Measurement Units"=w46:T7, "Meter 2.Measurement Units"=w47:T7, "Meter 1.Data Frame Format"=w45:T9, "Meter 2.Data Frame Format"=w44:T9)
    }
    frame "Meter Bank 2" {
      n3 = Unbundle By Name(w71) -> ("Meter 4.SLPM Error @ Zero"=w66:dbl, "Meter 3.SLPM Error @ Zero"=w65:dbl, "Meter 4.Meter Visa"=w70:refnum<visa-resource-name>, "Meter 4.Meter Present"=w67:bool, "Meter 3.Meter Visa"=w69:refnum<visa-resource-name>, "Meter 3.Meter Present"=w68:bool, "Meter Bank 2.Panel Data.Heating Value (BTU/ft³)"=w64:dbl, "Meter 3.Measurement Units"=w62:T7, "Meter 4.Measurement Units"=w61:T7, "Meter 3.Data Frame Format"=w60:T9, "Meter 4.Data Frame Format"=w59:T9)
    }
    frame "Meter Bank 3" {
      # "Use the selected Meter ID\nto determine the correct meter and\ninfo"
      n4 = Unbundle By Name(w86) -> ("Meter 6.SLPM Error @ Zero"=w80:dbl, "Meter 5.SLPM Error @ Zero"=w81:dbl, "Meter 6.Meter Visa"=w85:refnum<visa-resource-name>, "Meter 6.Meter Present"=w82:bool, "Meter 5.Meter Visa"=w84:refnum<visa-resource-name>, "Meter 5.Meter Present"=w83:bool, "Meter Bank 3.Panel Data.Heating Value (BTU/ft³)"=w79:dbl, "Meter 5.Measurement Units"=w77:T7, "Meter 6.Measurement Units"=w76:T7, "Meter 5.Data Frame Format"=w75:T9, "Meter 6.Data Frame Format"=w74:T9)
    }
  }
  n5 = flat-sequence {
    tunnel: "error in (no error)" -> [_]
    tunnel: [w89] -> w7
    frame #0 {
      n6 = Get Date/Time In Seconds() -> (seconds since 1Jan1904=w89:timestamp)
    }
  }
  n7 = call "FMA1600A Meter Present.vi"("Unit ID"=w13, "error in (no error)"="error in (no error)", "Meter Present"=w36, "Data Frame Format In"=w2, "VISA Refnum in"=w19) -> ("error out"=w9:errorcluster, "Data Cluster"=w14:T14)  [unwired: 4 in, 1 out]
  n8 = flat-sequence {
    tunnel: w9 -> [_]
    tunnel: [w90] -> w5
    frame #0 {
      n9 = Get Date/Time In Seconds() -> (seconds since 1Jan1904=w90:timestamp)
    }
  }
  n10 = Subtract(x=w5, y=w7) -> (x-y=→"x-y":dbl)
  n11 = call "FMA1600A Meter Present.vi"("Unit ID"=w12, "error in (no error)"=w9, "Meter Present"=w34, "Data Frame Format In"=w1, "VISA Refnum in"=w35) -> ("error out"=w8:errorcluster, "Data Cluster"=w11:T14)  [unwired: 4 in, 1 out]
  n12 = flat-sequence {
    tunnel: w8 -> [_]
    tunnel: [w91] -> w6
    frame #0 {
      n13 = Get Date/Time In Seconds() -> (seconds since 1Jan1904=w91:timestamp)
    }
  }
  n14 = case shown="1" w41 {
    tunnel: [w94 w101 w109 w127] -> w38
    tunnel: [w94 w100 w108 w126] -> w39
    tunnel: [w94 w99 w107 w125] -> w40
    tunnel: [w94 w98 w106 w124] -> w33
    tunnel: ["" ("Gas Type") w97 w105 w123] -> w25
    tunnel: [w94 w102 w110 w128] -> w23
    tunnel: w8 -> [w93 w104 w113 w122]
    tunnel: [w93 w104 w113 w121] -> w22
    tunnel: w21 -> [_ _ _ w120]
    tunnel: w20 -> [_ _ _ w119]
    tunnel: ["" ("Meter ID") w96 w112 w114] -> w18
    tunnel: w14 -> [_ w103 _ w118]
    tunnel: w13 -> [_ w96 _ w116]
    tunnel: w12 -> [_ _ w112 w115]
    tunnel: w11 -> [_ _ w111 w117]
    frame 0, Default {
      w94 = 0.0 ("Pressure (PSIA)")
      # "Disabled"
    }
    frame 1 {
      # "Meter 1,3,5"
      n15 = Unbundle By Name(w103) -> ("Totalizer"=w102:dbl, "Absolute Pressure"=w101:dbl, "Temperature"=w100:dbl, "Volumetric Flow"=w99:dbl, "Mass Flow"=w98:dbl, "Gas selected"=w97:string)
    }
    frame 2 {
      # "Meter 2,4,6"
      n16 = Unbundle By Name(w111) -> ("Totalizer"=w110:dbl, "Absolute Pressure"=w109:dbl, "Temperature"=w108:dbl, "Volumetric Flow"=w107:dbl, "Mass Flow"=w106:dbl, "Gas selected"=w105:string)
    }
    frame 3 {
      # "Auto"
      n17 = call "RANGE Auto Mode.vi"("Meter 246"=w115, "SLPM Error @ Zero (2,4,6)"=w119, "Meter 135"=w116, "SLPM Error @ Zero (1,3,5)"=w120, "Error In"=w122, "Meter 2,4,6"=w118, "Meter 1,3,5"=w117) -> ("Error Out"=w121:errorcluster, "Meter ID"=w114:string, "Output"=w129:T14)  [unwired: 1 in, 1 out]
      n18 = Unbundle By Name(w129) -> ("Totalizer"=w128:dbl, "Absolute Pressure"=w127:dbl, "Temperature"=w126:dbl, "Volumetric Flow"=w125:dbl, "Mass Flow"=w124:dbl, "Gas selected"=w123:string)
    }
  }
  n19 = Subtract(x=w6, y=w5) -> (x-y=→"x-y 2":dbl)
  n20 = case shown="\"D\"" w18 {
    tunnel: w17 -> [w130 _ w132 _ w134 _]
    tunnel: w16 -> [_ w131 _ w133 _ w135]
    tunnel: [w130 w131 w132 w133 w134 w135] -> w15
    frame "A", Default {
    }
    frame "B" {
    }
    frame "C" {
    }
    frame "D" {
    }
    frame "E" {
    }
    frame "F" {
    }
  }
  n21 = case shown="True" "Use Mass Flow Unit Converter?" {
    tunnel: w33 -> [w136 w143]
    tunnel: [w137 w141] -> w30
    tunnel: [w136 w140] -> w28
    tunnel: w22 -> [w137 w139]
    tunnel: w15 -> [_ w138]
    frame False {
    }
    frame True {
      n22 = call "RANGE Mass Flow Unit Conversion.vi"("Meter Units Out"=w138, "Ft³/HR -SLPM (T)"=FALSE, "Error In"=w139, "Input Mass Flow Rate"=w143) -> ("Error Out"=w141:errorcluster, "Output Mass Flow Rate"=w140:dbl)  [unwired: 6 in]
    }
  }
  n23 = call "RANGE General Factors.vi"("Error In"=w30, "Gas Type String"=w25) -> ("Error Out"=w31:errorcluster, "Flow Rate Factor"=w32:dbl)  [unwired: 8 in]
  n24 = call "RANGE Flow Rate Calculation.vi"("Error In"=w31, "Heating Value (BTU/ft³)"=w26, "Flow Rate Factor"=w32, "Ft³/HR"=w28) -> ("Error Out"=→"error out":errorcluster, "Flow Rate (BTU/Hr)"=w29:dbl)  [unwired: 6 in]
  n25 = case shown="\"Meter Bank 1\", Default" "Meter Number" {
    tunnel: "DAQ Data In in" -> [w157 w171 w185]
    tunnel: w38 -> [w156 w168 w184]
    tunnel: w39 -> [w155 w167 w183]
    tunnel: w40 -> [w154 w166 w182]
    tunnel: w33 -> [w153 w165 w181]
    tunnel: [w152 w170 w180] -> w43
    tunnel: w28 -> [w150 w164 w179]
    tunnel: w29 -> [w151 w163 w178]
    tunnel: w25 -> [w149 w162 w177]
    tunnel: w23 -> [w147 w161 w175]
    tunnel: w18 -> [w144 w158 w172]
    frame "Meter Bank 1", Default {
      n26 = call "RANGE Check For Totalizer.vi"("Calculated Totalizer"="Tot.Flow (Liters) Bank 1", "Meter Totalizer"=w147) -> ("Tot. Flow (Liters) out"=w146:dbl)  [unwired: 9 in]
      n27 = call "RANGE Check Standard Gas.vi"("Gas Type"=w149) -> ("Gas Type"=w148:string)  [unwired: 9 in, 1 out]
      n28 = Bundle By Name(cluster=w157, "Meter Bank 1.Meter ID"=w144, "Meter Bank 1.Panel Data.Tot.Flow"=w146, "Meter Bank 1.Panel Data.Gas Pressure"=w156, "Meter Bank 1.Panel Data.Gas Temperature"=w155, "Meter Bank 1.Panel Data.Vol. Flow"=w154, "Meter Bank 1.Panel Data.Mass Flow"=w153, "Meter Bank 1.Panel Data.Ft³ / Hr (SCFH)"=w150, "Meter Bank 1.Flow Rate (BTU/HR)"=w151, "Meter Bank 1.Panel Data.Meter Type (Gas)"=w148) -> (w152:T4)
    }
    frame "Meter Bank 2" {
      n29 = call "RANGE Check Standard Gas.vi"("Gas Type"=w162) -> ("Gas Type"=w169:string)  [unwired: 9 in, 1 out]
      n30 = call "RANGE Check For Totalizer.vi"("Calculated Totalizer"="Tot.Flow (Liters) Bank 2", "Meter Totalizer"=w161) -> ("Tot. Flow (Liters) out"=w160:dbl)  [unwired: 9 in]
      n31 = Bundle By Name(cluster=w171, "Meter Bank 2.Meter ID"=w158, "Meter Bank 2.Panel Data.Tot.Flow"=w160, "Meter Bank 2.Panel Data.Gas Pressure"=w168, "Meter Bank 2.Panel Data.Gas Temperature"=w167, "Meter Bank 2.Panel Data.Vol. Flow"=w166, "Meter Bank 2.Panel Data.Mass Flow"=w165, "Meter Bank 2.Panel Data.Ft³ / Hr (SCFH)"=w164, "Meter Bank 2.Flow Rate (BTU/HR)"=w163, "Meter Bank 2.Panel Data.Meter Type (Gas)"=w169) -> (w170:T4)
    }
    frame "Meter Bank 3" {
      n32 = call "RANGE Check Standard Gas.vi"("Gas Type"=w177) -> ("Gas Type"=w176:string)  [unwired: 9 in, 1 out]
      n33 = call "RANGE Check For Totalizer.vi"("Calculated Totalizer"="Tot.Flow (Liters) Bank 3", "Meter Totalizer"=w175) -> ("Tot. Flow (Liters) out"=w174:dbl)  [unwired: 9 in]
      n34 = Bundle By Name(cluster=w185, "Meter Bank 3.Meter ID"=w172, "Meter Bank 3.Panel Data.Tot.Flow"=w174, "Meter Bank 3.Panel Data.Gas Pressure"=w184, "Meter Bank 3.Panel Data.Gas Temperature"=w183, "Meter Bank 3.Panel Data.Vol. Flow"=w182, "Meter Bank 3.Panel Data.Mass Flow"=w181, "Meter Bank 3.Panel Data.Ft³ / Hr (SCFH)"=w179, "Meter Bank 3.Flow Rate (BTU/HR)"=w178, "Meter Bank 3.Panel Data.Meter Type (Gas)"=w176) -> (w180:T4)
    }
  }
  "DAQ Data In out" <- w43
